vi "Connect.vi"(8 "error in (no error)":errorcluster, 10 "Connection String":string, 11 "SqliteConnection in":refnum<class "DBC.lvclass">) -> (0 "error out":errorcluster, 3 "SqliteConnection out":refnum<class "DBC.lvclass">)   [LabVIEW 2020, in "ORM_DBC_Kdb.lvlib" / "DBC.lvclass"]
uses:
  DBC.lvclass
  C:/Program Files/National Instruments/LabVIEW 2020/vi.lib/Viviota/shared/ORM_DBC_dotNet.lvlibp/dbcDotNet/ORM_DBC_dotNet.lvclass
  C:/Program Files/National Instruments/LabVIEW 2020/vi.lib/Viviota/shared/ORM.lvlibp/ORM/DbConnection/DbConnection.lvclass
  C:/Viviota/Projects/R&D/__OpenSource/VIV_ORM/libraries/kdb/KpNet.KdbPlusClient.dll
  libraries/kdb/KpNet.KdbPlusClient.dll
  <vilib>/Viviota/shared/ORM_DBC_dotNet.lvlibp/dbcDotNet/Write connection.vi
  <vilib>/Viviota/shared/ORM.lvlibp/ORM/DbConnection/Write ColumnNameEqualsValueFormat.vi
  <vilib>/Viviota/shared/ORM.lvlibp/ORM/DbConnection/Write ColumnNameFormat.vi
  <vilib>/Viviota/shared/ORM.lvlibp/ORM/DbConnection/Write LastIdentityQuery.vi
  <vilib>/Viviota/shared/ORM.lvlibp/ORM/DbConnection/Write SupportTX.vi
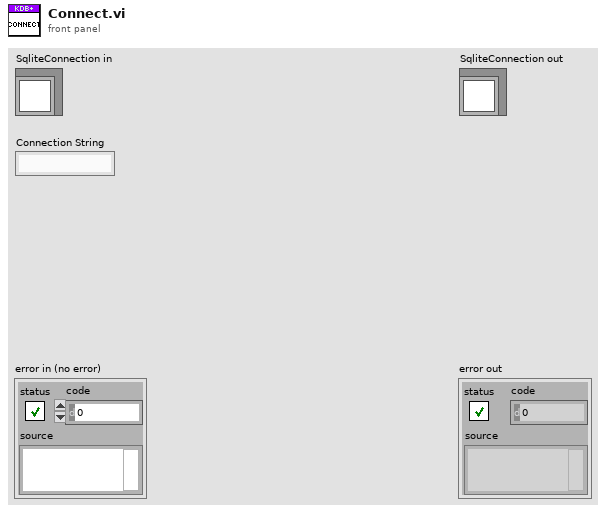
[diagram p1: front panel]
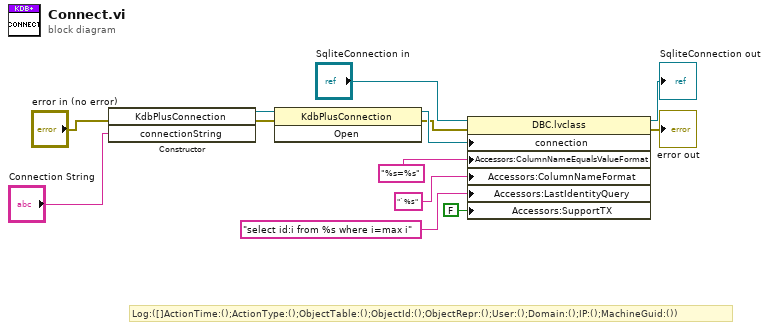
[diagram p0: block diagram]
diagram:
  # "Log:([]ActionTime:();ActionType:();ObjectTable:();ObjectId:();ObjectRepr:();User:();Domain:();IP:();MachineGuid:())"
  n1 = constructor class="KdbPlusConnection"(error in="error in (no error)", "connectionString"="Connection String") -> (reference out=w7:refnum<k24>, error out=w2:errorcluster)  [unwired: 2 in, 2 out]
  n2 = invoke class="KdbPlusConnection" method="Open"(reference=w7, error in=w2) -> (reference out=w6:refnum<k24>, error out=w1:errorcluster)  [unwired: 1 in, 1 out]
  n3 = property class="DBC.lvclass"(reference="SqliteConnection in", error in=w1, "connection"=w6, "Accessors:ColumnNameEqualsValueFormat"="%s=%s" ("ColumnNameFormat"), "Accessors:ColumnNameFormat"="`%s" ("ColumnNameFormat"), "Accessors:LastIdentityQuery"="select id:i from %s where i=max i" ("LastIdentityQuery"), "Accessors:SupportTX"=FALSE ("SupportTX")) -> (reference out=→"SqliteConnection out":refnum<class "DBC.lvclass">, error out=→"error out":errorcluster)
